vi "836_Camera Registry.vi"(8 "error in (no error)":errorcluster, 10 "Camera Address":string="192.168.0.90", 11 "Action":T2) -> (0 "error out":errorcluster, 3 "CameraDevRef":T1)   [LabVIEW 2015]
doc: "This software is licensed. Open the labview\\readme\\WPI Robotics Library Open Source License.txt file for more information."
uses:
  <vilib>/Rock Robotics/WPI/Camera/WPI_CameraRegistryActions.ctl
  <vilib>/Rock Robotics/WPI/Camera/WPI_CameraDevRef.ctl
  <vilib>/Rock Robotics/WPI/Camera/WPI_CameraSettings Operations.ctl
  <vilib>/Rock Robotics/WPI/Camera/WPI_CameraSettings Control.ctl
  <vilib>/Rock Robotics/SystemInterfaces/NetworkCommunication/NetComm_UsageReport_ResourceType.ctl
  <vilib>/vision/driver/NI_Vision_Acquisition_Software.lvlib
panel:
  out "Camera Addresses":string[](array[string])
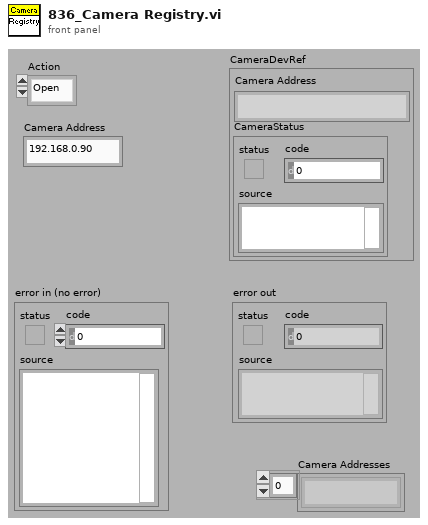
[diagram p1: front panel]
types:
  T1 = typedef "WPI_CameraDevRef.ctl" = cluster{"Camera Address":string, "CameraStatus":errorcluster}
  T2 = typedef "WPI_CameraRegistryActions.ctl" = enum16{"Open", "Close"}
  T3 = typedef "WPI_CameraSettings Control.ctl" = cluster{"FPS":i32, "Compression":i32, "Size":i32, "White Balance":i32, "Brightness":i32, "Sharpness":i32, "Exposure":i32, "Color Level":i32, "Exposure Priority":i32, "Color Enable":i32, "JPG Loop":i32, "MJPG Loop":i32, "Exposure Value":i32}
  T4 = typedef "WPI_CameraSettings Operations.ctl" = enum16{"Udate FPS", "Update Compression", "Update Size", "Update White Balance", "Update Brightness", "Update Sharpness", "Update Exposure", "Update Exposure Value", "Update Color Level", "Update Exp Priority", "Update Color Enable", "Update JPG", "Update MJPG", "Read and Clear", "Read", "Init"}
  T5 = typedef "NetComm_UsageReport_ResourceType.ctl" = enum8{"Controller", "Module", "Language", "CANPlugin", "Accelerometer", "ADXL345", "AnalogChannel", "AnalogTrigger", "AnalogTriggerOutput", "CANJaguar", "Compressor", "Counter", "Dashboard", "DigitalInput", "DigitalOutput", "DriverStationCIO", "DriverStationEIO", "DriverStationLCD", "Encoder", "GearTooth", "Gyro", "I2C", "Framework", "Jaguar", "Joystick", "Kinect", "KinectStick", "PIDController", "Preferences", "PWM", "Relay", "RobotDrive", "SerialPort", "Servo", "Solenoid", "SPI", "Task", "Ultrasonic", "Victor", "Button", "Command", "AxisCamera", "PCVideoServer", "SmartDashboard", "Talon", "HiTechnicColorSensor", "HiTechnicAccel", "HiTechnicCompass", "SRF08", "AnalogOutput", "Victor SP", "Talon SRX", "CAN Talon SRX", "ADXL362 Accel", "ADXRS450 Gyro", "Rev SPARK", "Mindsensors SD540", "Digital Filter"}
  T6 = typedef "WPI_CameraImageSize.ctl" = enum16{"640x480", "320x240", "160x120", "Custom"}
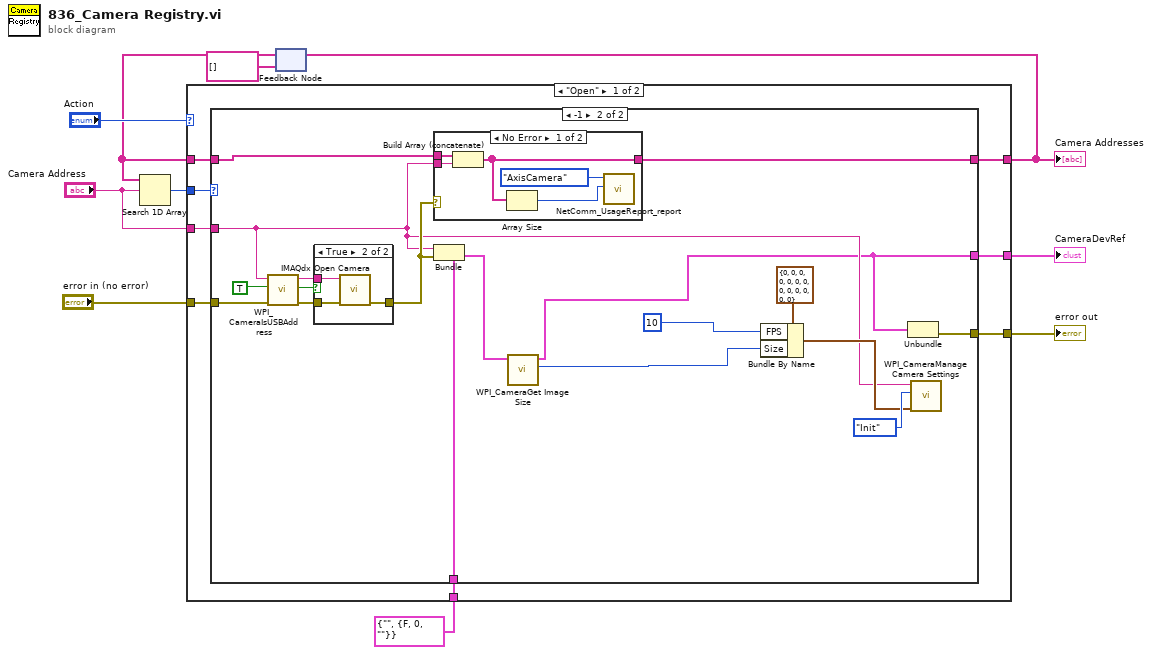
[diagram p0: block diagram]
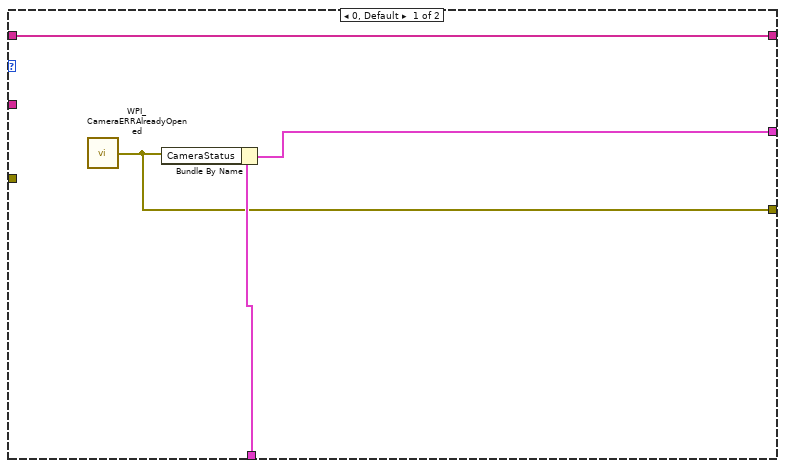
[diagram p2: hidden frame]
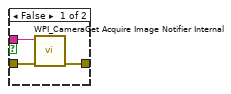
[diagram p3: hidden frame]
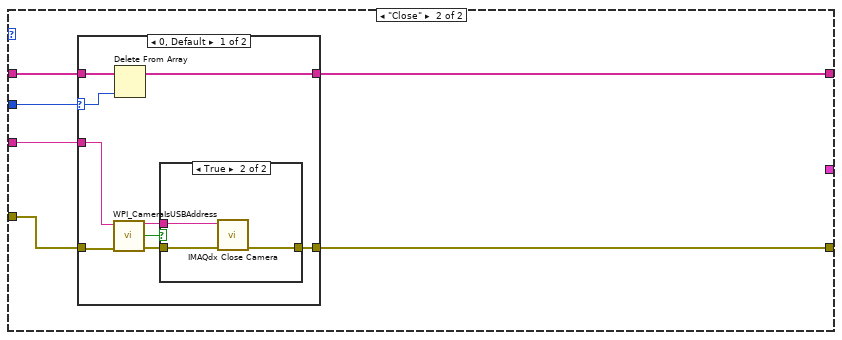
[diagram p5: hidden frame]
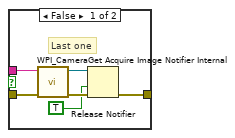
[diagram p6: hidden frame]
diagram:
  n1 = feedback #1(string[] []) -> (w4:string[])
  n2 = Search 1D Array(1D array=w4, element="Camera Address") -> (index of element=w5:i32)  [unwired: 1 out]
  n3 = case shown="\"Open\"" "Action" {
    tunnel: w4 -> [w17 w57]
    tunnel: "Camera Address" -> [w18 w53]
    tunnel: [w16 _] -> w9
    tunnel: w5 -> [w15 w58]
    tunnel: [w14 w56] -> w6
    tunnel: "error in (no error)" -> [w13 w55]
    tunnel: [w12 w54] -> w7
    tunnel: T1 {"Camera Address"="", "CameraStatus"={"status"=FALSE, "code"=0, "source"=""}} ("CameraDevRef") -> [w11 _]
    frame "Open" {
      n4 = case shown="-1" w15 {
        tunnel: w18 -> [_ w26]
        tunnel: w17 -> [w22 w40]
        tunnel: [w19 w24] -> w16
        tunnel: [w22 w39] -> w14
        tunnel: w13 -> [_ w32]
        tunnel: [w20 w27] -> w12
        tunnel: w11 -> [w21 w38]
        frame 0, Default {
          n5 = call <vilib>:"WPI_CameraERRAlreadyOpened.vi"() -> ("error out"=w20:errorcluster)
          n6 = Bundle By Name(cluster=w21, "CameraStatus"=w20) -> (w19:T1)
        }
        frame -1 {
          n7 = call <vilib>:"WPI_CameraIsUSBAddress.vi"("error in (no error)"=w32, "Enumerate?"=TRUE, "Camera Address In"=w26) -> ("error out"=w31:errorcluster, "USB?"=w29:bool, "Camera Address Out"=w30:string)  [unwired: 6 in]
          n8 = case shown="True" w29 {
            tunnel: [w43 w45] -> w36
            tunnel: w31 -> [w42 w46]
            tunnel: w30 -> [w41 w44]
            frame False {
              n9 = call <vilib>:"WPI_CameraGet Acquire Image Notifier Internal.vi"("error in (no error)"=w42, "Camera Address"=w41) -> ("error out"=w43:errorcluster)  [unwired: 9 out]
            }
            frame True {
              n10 = call <vilib>:"IMAQdx Open Camera.vi"("error in"=w46, "Session In"=w44) -> ("error out"=w45:errorcluster)  [unwired: 8 in, 1 out]
            }
          }
          n11 = case shown="No Error" w36 {
            tunnel: w40 -> [w51 w52]
            tunnel: w26 -> [w50 _]
            tunnel: [w48 w52] -> w39
            frame No Error {
              n12 = Build Array (concatenate)(w51, w50) -> (w48:string[])
              n13 = Array Size(array=w48) -> (size(s)=w47:i32)
              n14 = call <vilib>:"NetComm_UsageReport_report.vi"("Instance Number"=w47, "Resource Type"=NetComm_UsageReport_ResourceType."AxisCamera") -> ()  [unwired: 10 in]
            }
            frame Error {
            }
          }
          n15 = Bundle(cluster=w38, "Camera Address"=w26, "CameraStatus"=w36) -> (w25:T1)
          n16 = call <vilib>:"WPI_CameraGet Image Size.vi"("CameraDevRef"=w25) -> ("Image Size"=w23:T6, "CameraDevRef Out"=w24:T1)  [unwired: 7 in, 2 out]
          n17 = Bundle By Name(cluster=T3 {"FPS"=0, "Compression"=0, "Size"=0, "White Balance"=0, "Brightness"=0, "Sharpness"=0, "Exposure"=0, "Color Level"=0, "Exposure Priority"=0, "Color Enable"=0, "JPG Loop"=0, "MJPG Loop"=0, "Exposure Value"=0} ("Values In"), "FPS"=10, "Size"=w23) -> (w33:T3)
          n18 = Unbundle(w24) -> ("CameraStatus"=w27:errorcluster)  [unwired: 1 out]
          n19 = call <vilib>:"WPI_CameraManage Camera Settings.vi"("Values In"=w33, "Operation"=WPI_CameraSettings_Operations."Init", "Camera IP"=w26) -> ()  [unwired: 7 in, 2 out]
        }
      }
    }
    frame "Close" {
      n20 = case shown="0, Default" w58 {
        selector: w58 -> [w64 _]
        tunnel: w57 -> [w67 w78]
        tunnel: [w66 w78] -> w56
        tunnel: w55 -> [w62 w77]
        tunnel: [w65 w77] -> w54
        tunnel: w53 -> [w61 _]
        frame 0, Default {
          n21 = call <vilib>:"WPI_CameraIsUSBAddress.vi"("error in (no error)"=w62, "Camera Address In"=w61) -> ("error out"=w63:errorcluster, "USB?"=w59:bool, "Camera Address Out"=w60:string)  [unwired: 7 in]
          n22 = Delete From Array(array=w67, index=w64) -> (array with subset deleted=w66:string[])  [unwired: 1 in, 1 out]
          n23 = case shown="True" w59 {
            tunnel: w63 -> [w73 w75]
            tunnel: [w72 w74] -> w65
            tunnel: w60 -> [w68 w76]
            frame False {
              # "Last one"
              n24 = call <vilib>:"WPI_CameraGet Acquire Image Notifier Internal.vi"("error in (no error)"=w73, "Camera Address"=w68) -> ("error out"=w71:errorcluster, "Acquire Image Notifier"=w70:refnum<notifier>)  [unwired: 8 out]
              n25 = Release Notifier(notifier=w70, force destroy? (F)=TRUE, error in (no error)=w71) -> (error out=w72:errorcluster)  [unwired: 2 out]
            }
            frame True {
              n26 = call <vilib>:"IMAQdx Close Camera.vi"("error in"=w75, "Session In"=w76) -> ("error out"=w74:errorcluster)  [unwired: 9 in]
            }
          }
        }
        frame -1 {
        }
      }
    }
  }
  "CameraDevRef" <- w9
  "error out" <- w7
  "Camera Addresses" <- w6
  n27 = feedback-in #1(w6) -> ()
